vi "Tree+InfoString+Graph.vi"() -> ()   [LabVIEW 2013]
panel:
  in  "Select Page Tree":string(tree)
  out "波形图":dbl[](graph)
  out "Status":string
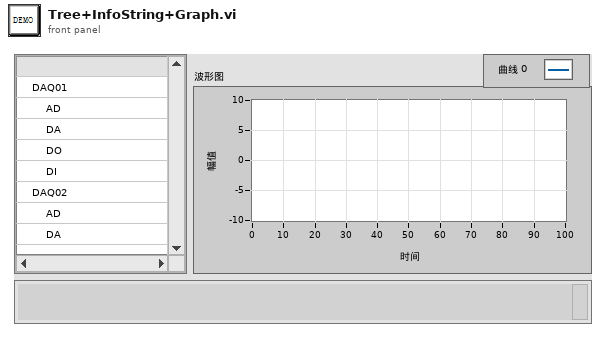
[diagram p1: front panel]
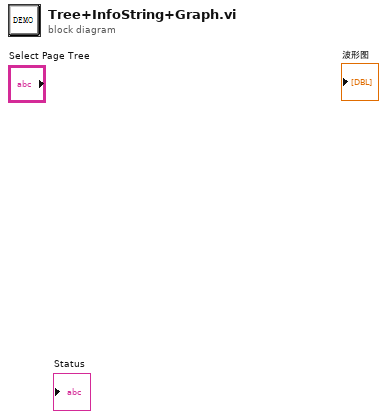
[diagram p0: block diagram]
diagram:
